vi "CreateScanListNode.vi"(7 "DOM Document":refnum<k20>, 8 "Error In":errorcluster, 11 "Scan List":string) -> (0 "Error Out":errorcluster, 3 "Scan List Node":refnum<k20>)   [LabVIEW 2012]
uses:
  libs/LV-Utilities/LV-Utilities.lvlib
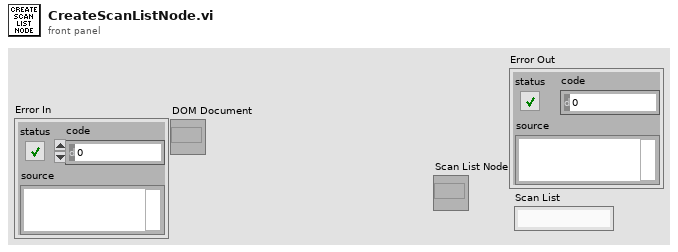
[diagram p1: front panel]
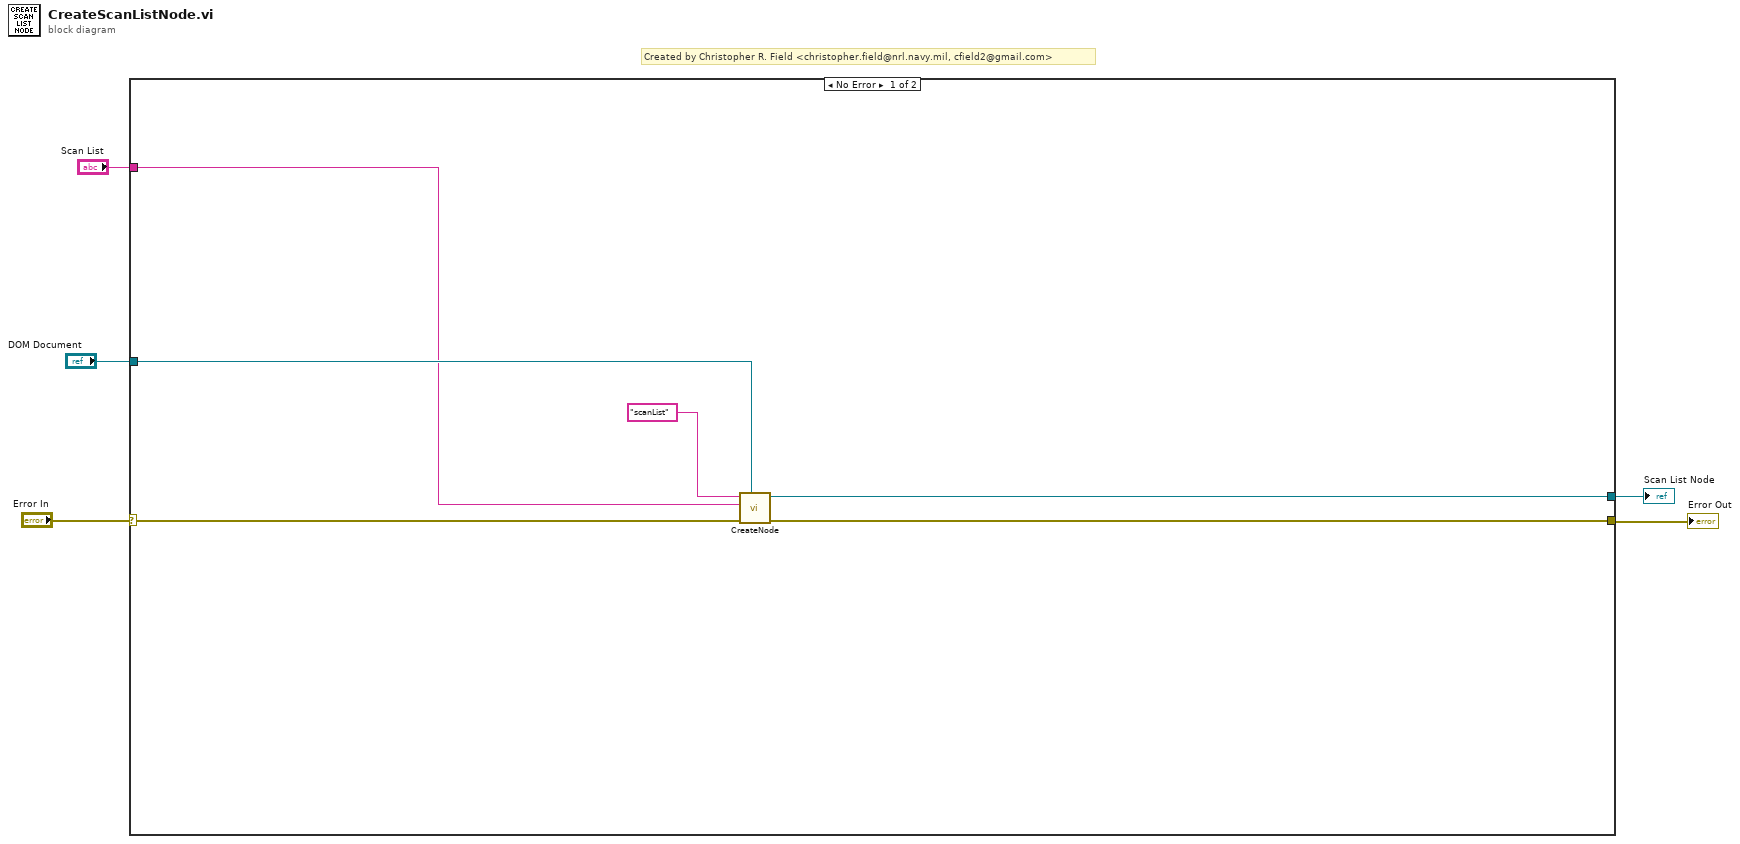
[diagram p0: block diagram]
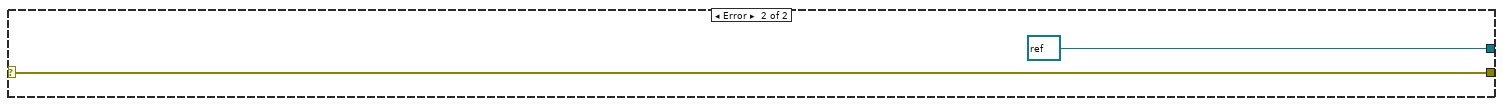
[diagram p2: hidden frame]
diagram:
  # "Created by Christopher R. Field <christopher.field@nrl.navy.mil, cfield2@gmail.com>"
  n1 = case shown="No Error" "Error In" {
    selector: "Error In" -> [w11 w13]
    tunnel: "DOM Document" -> [w9 _]
    tunnel: [w7 w13] -> w3
    tunnel: "Scan List" -> [w8 _]
    tunnel: [w6 refnum<k20> refnum ("Wirings Node 2")] -> w1
    frame No Error {
      n2 = call "CreateNode.vi"("DOM Document"=w9, "Error In"=w11, "Text"=w8, "Tag Name"="scanList") -> ("Error out"=w7:errorcluster, "Node"=w6:refnum<k20>)  [unwired: 6 in]
    }
    frame Error {
    }
  }
  "Scan List Node" <- w1
  "Error Out" <- w3
